vi "Round.vi"(11 "Team in":refnum<class "Team.lvclass">) -> (2 "Round":u32)   [LabVIEW 2020, in "SquareBattle.lvlib" / "Team.lvclass"]
uses:
  Team.lvclass
  Team.lvclass/Team.ctl
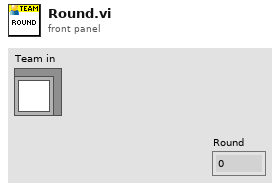
[diagram p1: front panel]
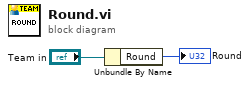
[diagram p0: block diagram]
diagram:
  n1 = Unbundle By Name("Team in") -> ("Round"=→"Round":u32)
